vi "tsc--Determine Dominant Color.vi"(8 "error in":errorcluster, 11 "orig file":path) -> (0 "error out":errorcluster, 2 "maximum color":u32(colorbox), 3 "orig file out":path)   [LabVIEW 2021, in "Material SubVIs.lvlib"]
doc: "Find the dominant color from the existing image.\n\n<b>Note</b>: Assumes a single color PNG file\n\n<b>Note</b>: Uses <i>System.Drawing</i> .NET functionality\n\n<b>Code Developed By:</b> +\nDaniel Coons +\nTechnology Service Corporation +\nwww.tsc.com/atcs"
uses:
  Material SubVIs.lvlib
  System.Drawing
panel:
  out "Map":map{u32, i32}(c390)
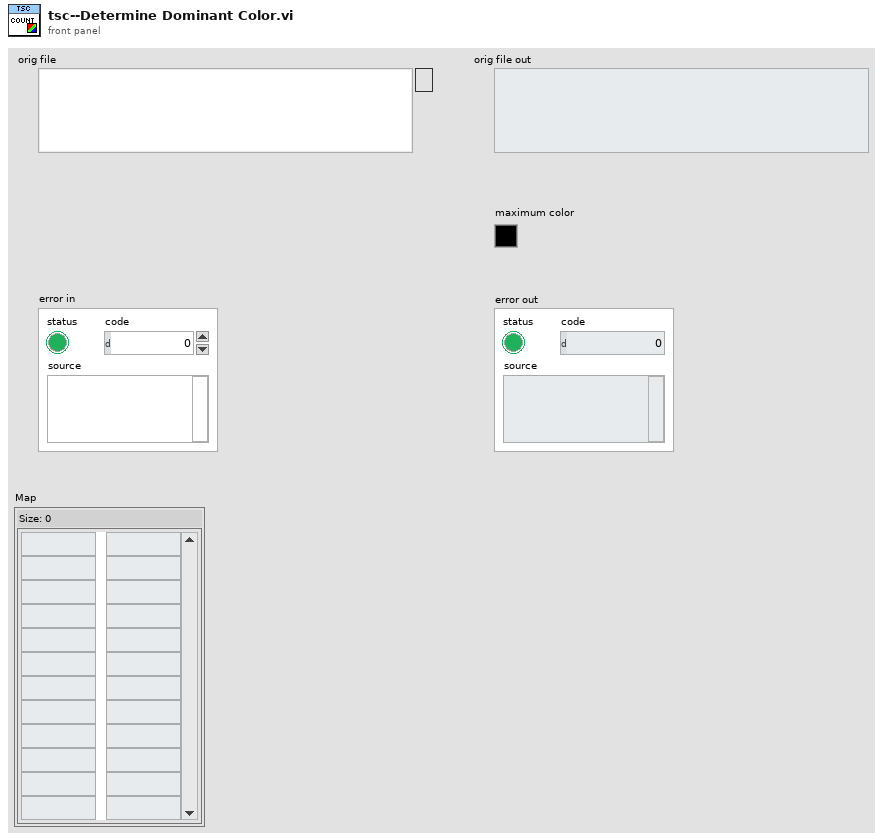
[diagram p1: front panel]
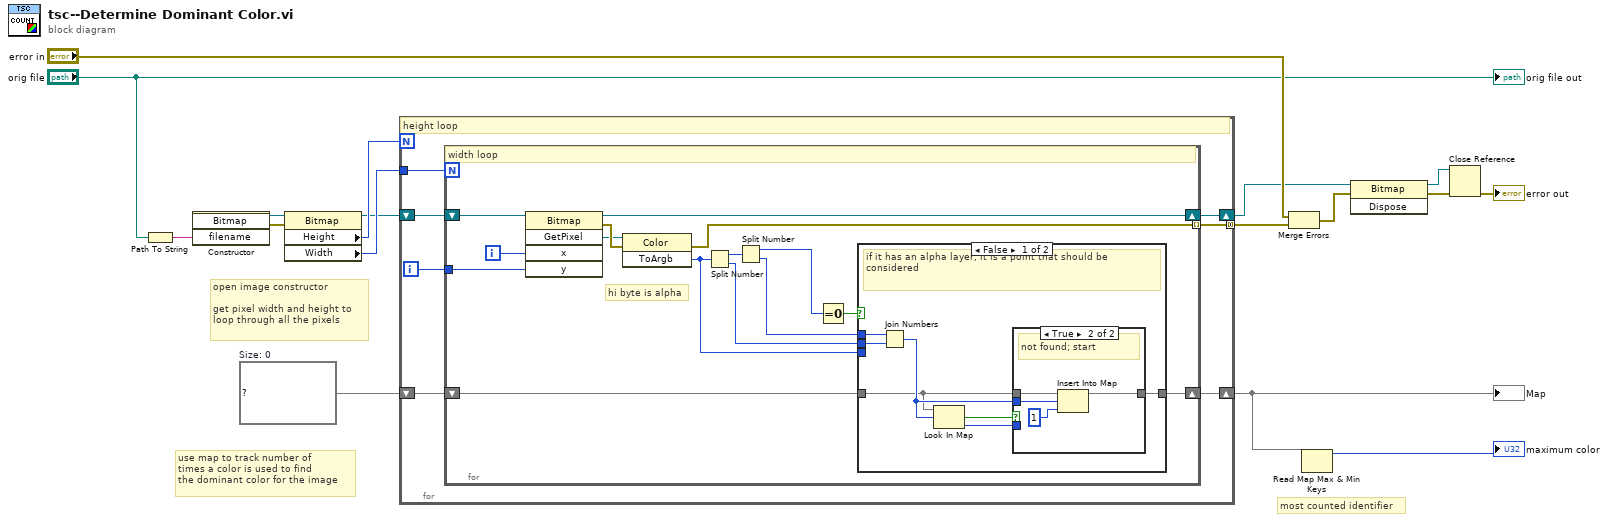
[diagram p0: block diagram]
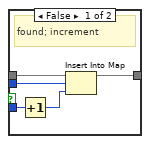
[diagram p2: hidden frame]
diagram:
  w5 = map{u32, i32} {}  # Size: 0
  # "most counted identifier"
  # "use map to track number of\ntimes a color is used to find\nthe dominant color for the image"
  # "open image constructor\n\nget pixel width and height to \nloop through all the pixels"
  n1 = Path To String(path="orig file") -> (string=w12:string)
  n2 = constructor class="Bitmap"("filename"=w12) -> (reference out=w11:refnum<k24>, error out=w13:errorcluster)  [unwired: 3 in, 2 out]
  n3 = property class="Bitmap"(reference=w11, error in=w13) -> (reference out=w8:refnum<k24>, "Height"=w10:i32, "Width"=w9:i32)  [unwired: 1 out]
  n4 = for {
    N: w10 -> [_]
    tunnel: w9 -> [w24]
    shift-right: [w21] -> w2
    shift-left: w8 -> [w22]
    tunnel: [w20] -> w7 mode=concatenating
    shift-right: [w18] -> w4
    shift-left: w5 -> [w19]
    i -> [w23]
    # "height loop"
    n5 = for {
      N: w24 -> [_]
      tunnel: w23 -> [w33]
      shift-right: [w35] -> w21
      shift-left: w22 -> [w36]
      tunnel: [w38] -> w20 mode=indexing
      shift-right: [w26] -> w18
      shift-left: w19 -> [w27]
      i -> [w34]
      # "hi byte is alpha"
      # "width loop"
      n6 = invoke class="Bitmap" method="GetPixel"(reference=w36, "x"=w34, "y"=w33) -> (reference out=w35:refnum<k24>, error out=w39:errorcluster, "GetPixel"=w37:refnum<k24>)  [unwired: 2 in, 2 out]
      n7 = invoke class="Color" method="ToArgb"(reference=w37, error in=w39) -> (error out=w38:errorcluster, "ToArgb"=w31:i32)  [unwired: 1 in, 1 out]
      n8 = Split Number(x=w31) -> (hi(x)=w29:u16, lo(x)=w30:u16)
      n9 = Split Number(x=w29) -> (hi(x)=w25:u8, lo(x)=w28:u8)
      n10 = Equal To 0?(x=w25) -> (x = 0?=w32:bool)
      n11 = case shown="False" w32 {
        tunnel: w31 -> [_ _]
        tunnel: w30 -> [w46 _]
        tunnel: w28 -> [w45 _]
        tunnel: w27 -> [w40 w56]
        tunnel: [w42 w56] -> w26
        frame False {
          # "if it has an alpha layer, it is a point that should be considered"
          n12 = Join Numbers(hi=w45, lo=w46) -> ((hi.lo)=w41:u32)
          n13 = Look In Map(map=w40, key=w41) -> (key not found?=w43:bool, value=w44:i32)  [unwired: 1 in]
          n14 = case shown="True" w43 {
            tunnel: w40 -> [w51 w55]
            tunnel: w41 -> [w50 w54]
            tunnel: w44 -> [w49 _]
            tunnel: [w47 w52] -> w42
            frame False {
              # "found; increment"
              n15 = Increment(x=w49) -> (x+1=w48:i32)
              n16 = Insert Into Map(map in=w51, key=w50, value=w48) -> (map out=w47:map{u32, i32})  [unwired: 2 out]
            }
            frame True {
              # "not found; start"
              n17 = Insert Into Map(map in=w55, key=w54, value=1) -> (map out=w52:map{u32, i32})  [unwired: 2 out]
            }
          }
        }
        frame True {
          # "no alpha, ignore"
        }
      }
    }
  }
  "Map" <- w4
  n18 = Merge Errors("error in", w7) -> (w17:errorcluster)
  n19 = Read Map Max & Min Keys(11:w4) -> (3:→"maximum color":u32)  [unwired: 1 out]
  n20 = invoke class="Bitmap" method="Dispose"(reference=w2, error in=w17) -> (reference out=w1:refnum<k24>, error out=w15:errorcluster)  [unwired: 1 in, 1 out]
  n21 = Close Reference(reference=w1, error in (no error)=w15) -> (error out=→"error out":errorcluster)
  "orig file out" <- "orig file"
